vi "New__slk_mt.vi"(8 "error in (no error)":errorcluster, 11 "wire refnum in":refnum<vi>) -> (0 "error out":errorcluster, 3 "wire out":refnum<class "Wire__slk_mt.lvclass">)   [LabVIEW 2013, in "Lazyboots Menu Tool.lvlib" / "Wire__slk_mt.lvclass"]
doc: "Creates new wire object by wire refnum."
uses:
  Wire__slk_mt.lvclass
  Segment/Segment__slk_mt.lvclass
panel:
  # "New__slk_mt.vi\nCreates new wire object by wire refnum.\n\nNOTICE -- YOU MUST LEAVE THIS NOTICE IN PLACE.\n\nCopyright (c) 2011, LIANG LIU Shawn.Liu.cn@gmail.com\nAll rights reserved.\n\nRedistribution and use in source and binary forms, with or without modification, are permitted provided that the following conditions are met:\n-Redistributions of source code must retain the above copyright notice, this list of conditions and the following disclaimer.\n-Redistributions in binary form must reproduce the above copyright notice, this list of conditions and the following disclaimer in the documentation and/or other materials provided with the distribution.\n-Neither the name of the eLp nor the names of its contributors may be used to endorse or promote products derived from this software without specific prior written permission.\n\nTHIS SOFTWARE IS PROVIDED BY THE COPYRIGHT HOLDERS AND CONTRIBUTORS \"AS IS\" AND ANY EXPRESS OR IMPLIED WARRANTIES, INCLUDING, BUT NOT LIMITED TO, THE IMPLIED WARRANTIES OF MERCHANTABILITY AND FITNESS FOR A PARTICULAR PURPOSE ARE DISCLAIMED. IN NO EVENT SHALL THE COPYRIGHT HOLDER OR CONTRIBUTORS BE LIABLE FOR ANY DIRECT, INDIRECT, INCIDENTAL, SPECIAL, EXEMPLARY, OR CONSEQUENTIAL DAMAGES (INCLUDING, BUT NOT LIMITED TO, PROCUREMENT OF SUBSTITUTE GOODS OR SERVICES; LOSS OF USE, DATA, OR PROFITS; OR BUSINESS INTERRUPTION) HOWEVER CAUSED AND ON ANY THEORY OF LIABILITY, WHETHER IN CONTRACT, STRICT LIABILITY, OR TORT (INCLUDING NEGLIGENCE OR OTHERWISE) ARISING IN ANY WAY OUT OF THE USE OF THIS SOFTWARE, EVEN IF ADVISED OF THE POSSIBILITY OF SUCH DAMAGE."
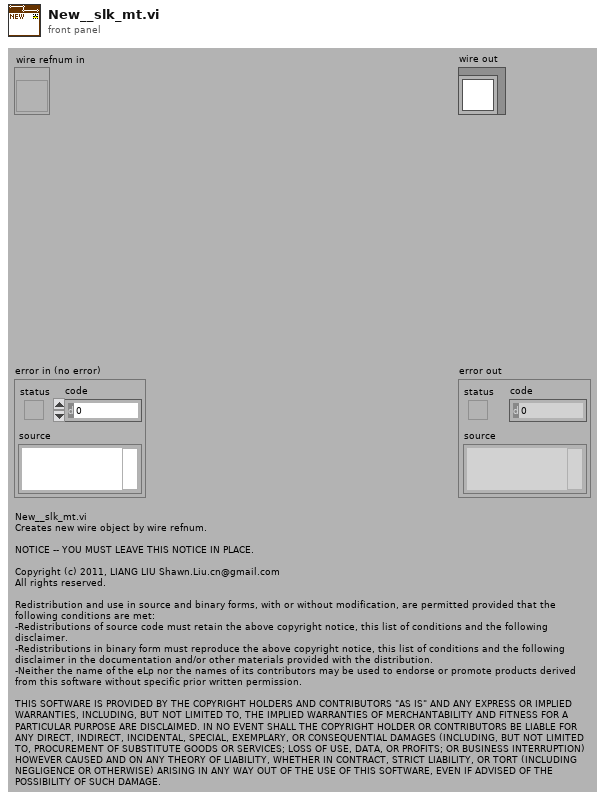
[diagram p1: front panel]
types:
  T1 = cluster{"Position":cluster{"h":i16, "v":i16}, "Flags":i32, "Type":enum32{"LooseEnd", "Endpoint", "Bend", "Junction"}, "Up Joint Index":i16, "Down Joint Index":i16, "Left Joint Index":i16, "Right Joint Index":i16}[]
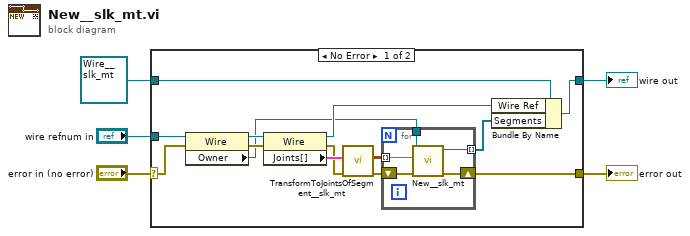
[diagram p0: block diagram]
diagram:
  n1 = case shown="No Error" "error in (no error)" {
    selector: "error in (no error)" -> [w14 w26]
    tunnel: [w13 w26] -> w4
    tunnel: [w18 w25] -> w2
    tunnel: refnum<class "Wire__slk_mt.lvclass"> refnum ("wire in") -> [w19 w25]
    tunnel: "wire refnum in" -> [w16 _]
    frame No Error {
      n2 = property class="Wire"(reference=w16, error in=w14) -> (reference out=w11:refnum<vi>, error out=w10:errorcluster, "Owner"=w6:refnum<vi>)
      n3 = property class="Wire"(reference=w11, error in=w10) -> (reference out=w7:refnum<vi>, error out=w8:errorcluster, "Joints[]"=w9:T1)
      n4 = call "TransformToJointsOfSegment__slk_mt.vi"("error in (no error)"=w8, "joints[]"=w9) -> ("error out"=w17:errorcluster, "joints[]"=w12:cluster{"X":i32, "Y":i32}[][])  [unwired: 8 in]
      n5 = for {
        shift-right: [w22] -> w13
        shift-left: w17 -> [w24]
        tunnel: [w23] -> w15 mode=indexing
        tunnel: w12 -> [w21] mode=indexing
        tunnel: w6 -> [w20]
        n6 = call "New__slk_mt.vi"("error in (no error)"=w24, "joints"=w21, "owner refnum in"=w20) -> ("error out"=w22:errorcluster, "segment out"=w23:refnum<class "Segment__slk_mt.lvclass">)  [unwired: 7 in]
      }
      n7 = Bundle By Name(cluster=w19, "Wire Ref"=w7, "Segments"=w15) -> (w18:refnum<class "Wire__slk_mt.lvclass">)
    }
    frame Error {
    }
  }
  "error out" <- w4
  "wire out" <- w2
